vi "GOOP_MyComputer_Interface_CreateNewWizard_IncludeItem.vi"(11 "Wizard":u64) -> (3 "Include me":bool)   [LabVIEW 2020]
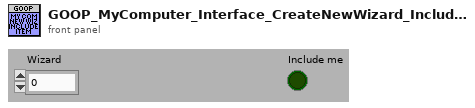
[diagram p1: front panel]
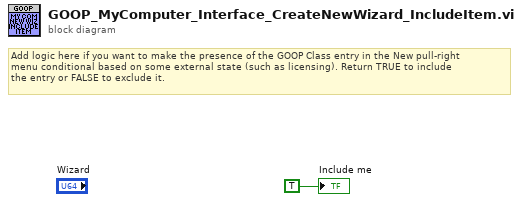
[diagram p0: block diagram]
diagram:
  # "Add logic here if you want to make the presence of the GOOP Class entry in the New pull-right\nmenu conditional based on some external state (such as licensing). Return TRUE to include\nthe entry or FALSE to exclude it."
  "Include me" <- TRUE ("Include me")
